vi "LRMS_Switching_Config.vi"(8 "error in (no error)":errorcluster, 11 "Sense MUX Devices":refnum<k15>[](array[refnum])) -> (0 "error out":errorcluster, 3 "Array":refnum<k15>[](array[refnum]))   [LabVIEW 2019]
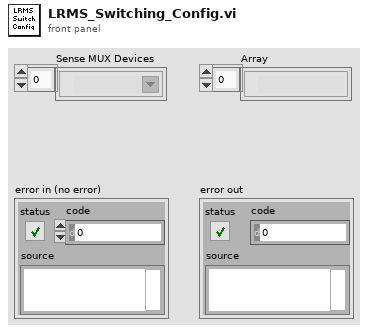
[diagram p1: front panel]
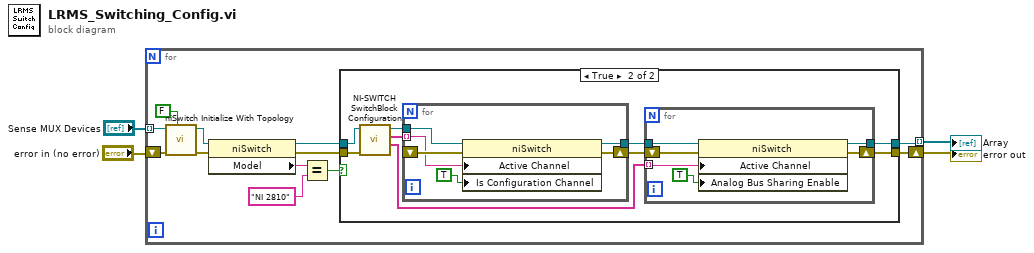
[diagram p0: block diagram]
diagram:
  n1 = for {
    tunnel: "Sense MUX Devices" -> [w16] mode=indexing
    shift-right: [w6] -> w3
    shift-left: "error in (no error)" -> [w14]
    tunnel: [w5] -> w4 mode=indexing
    n2 = call <instrlib>:"niSwitch Initialize With Topology.vi"("simulate (boolean value)"=FALSE, "error in (no error)"=w14, "resource name"=w16) -> ("error out"=w12:errorcluster, "instrument handle out"=w13:refnum<k15>)  [unwired: 7 in]
    n3 = property class="niSwitch"(reference=w13, error in=w12) -> (reference out=w10:refnum<k15>, error out=w11:errorcluster, "Model"=w9:string)
    n4 = Equal?(x=w9, y="NI 2810") -> (x = y?=w7:bool)
    n5 = case shown="True" w7 {
      tunnel: [w18 w24] -> w5
      tunnel: [w17 w23] -> w6
      tunnel: w11 -> [w17 w21]
      tunnel: w10 -> [w18 w20]
      frame False {
      }
      frame True {
        n6 = call "NI-SWITCH SwitchBlock Configuration.vi"("error in (no error)"=w21, "Reference In"=w20) -> ("Analog Bus Array"=w19:string[], "Row Array"=w26:string[], "Reference out"=w22:refnum<k15>)  [unwired: 6 in, 1 out]
        n7 = for {
          tunnel: w26 -> [w36] mode=indexing
          shift-right: [w38] -> w25
          shift-left: _ -> [w37]
          tunnel: w22 -> [w35]
          tunnel: [w34] -> w27
          n8 = property class="niSwitch"(reference=w35, error in=w37, "Active Channel"=w36, "Is Configuration Channel"=TRUE ("Channel Configuration:Is Configuration Channel")) -> (reference out=w34:refnum<k15>, error out=w38:errorcluster)
        }
        n9 = for {
          shift-right: [w30] -> w23
          shift-left: w25 -> [w31]
          tunnel: w27 -> [w32]
          tunnel: [w29] -> w24
          tunnel: w19 -> [w28] mode=indexing
          n10 = property class="niSwitch"(reference=w32, error in=w31, "Active Channel"=w28, "Analog Bus Sharing Enable"=TRUE ("Channel Configuration:Is Configuration Channel")) -> (reference out=w29:refnum<k15>, error out=w30:errorcluster)
        }
      }
    }
  }
  "Array" <- w4
  "error out" <- w3
